vi "Read Key I32.vi"(6 "Default Val":i32, 7 "Section Name":string, 8 "error in (no error)":errorcluster, 10 "Key Names":string, 11 "Config Data":T1(array[cluster])) -> (0 "error out":errorcluster, 1 "Key Names":string[](array[string]), 2 "Key Value out":i32, 3 "Config Data dup":T1(array[cluster]), 4 "Key Find?":bool)   [LabVIEW 2020, in "GUCalibration2.lvlib"]
uses:
  GUCalibration2.lvlib
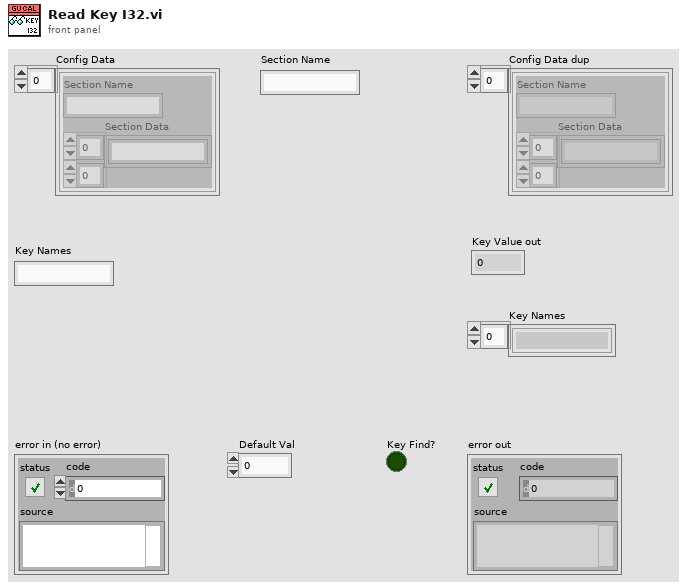
[diagram p1: front panel]
types:
  T1 = cluster{"Section Name":string, "Section Data":string[][]}[]
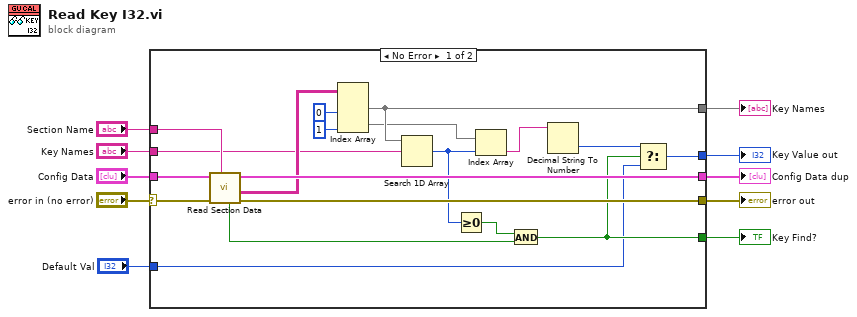
[diagram p0: block diagram]
diagram:
  n1 = case shown="No Error" "error in (no error)" {
    selector: "error in (no error)" -> [w27 w31]
    tunnel: "Section Name" -> [w28 _]
    tunnel: "Config Data" -> [w29 w30]
    tunnel: [w21 w31] -> w7
    tunnel: [w26 w30] -> w6
    tunnel: [w23 _] -> w5
    tunnel: "Key Names" -> [w22 _]
    tunnel: [w14 _] -> w3
    tunnel: "Default Val" -> [w12 _]
    tunnel: [w11 _] -> w1
    frame No Error {
      n2 = call "Read Section Data.vi"("Section Name"=w28, "error in (no error)"=w27, "Config Data"=w29) -> ("error out"=w21:errorcluster, "Section Data"=w25:string[][], "Config Data out"=w26:T1, "Section Exist"=w16:bool)  [unwired: 4 in, 1 out]
      n3 = Index Array(array=w25, index (col) #1=0 ("disabled index (col)"), index (col) #2=1 ("index (col)")) -> (element #1=w23:string[], element #2=w19:string[])  [unwired: 2 in]
      n4 = Search 1D Array(1D array=w23, element=w22) -> (index of element=w18:i32)  [unwired: 1 in]
      n5 = Greater Or Equal To 0?(x=w18) -> (x >= 0?=w17:bool)
      n6 = Index Array(array=w19, index=w18) -> (element=w15:string)
      n7 = And(x=w17, y=w16) -> (x .and. y?=w14:bool)
      n8 = Decimal String To Number(string=w15) -> (number=w13:i32)  [unwired: 2 in, 1 out]
      n9 = Select(t=w13, s=w14, f=w12) -> (s? t:f=w11:i32)
    }
    frame Error {
    }
  }
  "error out" <- w7
  "Key Names" <- w5
  "Config Data dup" <- w6
  "Key Find?" <- w3
  "Key Value out" <- w1
